vi "Interface.vi"(8 "error in (no error)":errorcluster, 11 "Display Image in":refnum<class "Display Image.lvclass">) -> (0 "error out":errorcluster, 3 "Display Image out":refnum<class "Display Image.lvclass">)   [LabVIEW 2018, in "Display Image.lvclass"]
doc: "This VI presents the interface to view the image acquired by the CCD."
uses:
  Display Image.lvclass
  <vilib>/Utility/inputDevices.llb/mouseAcquire.vi
panel:
  in  "Stop Button":bool
  out "Data:":dbl
  out "Y:":u16
  out "X:":u16
  in  "Histogram":bool
  in  "Logarithmic":bool
  in  "Linear":bool
  out "Stddev":dbl
  out "Mean":dbl
  out "Intensity Graph":dbl[][](graph)
  # "Image Graph"
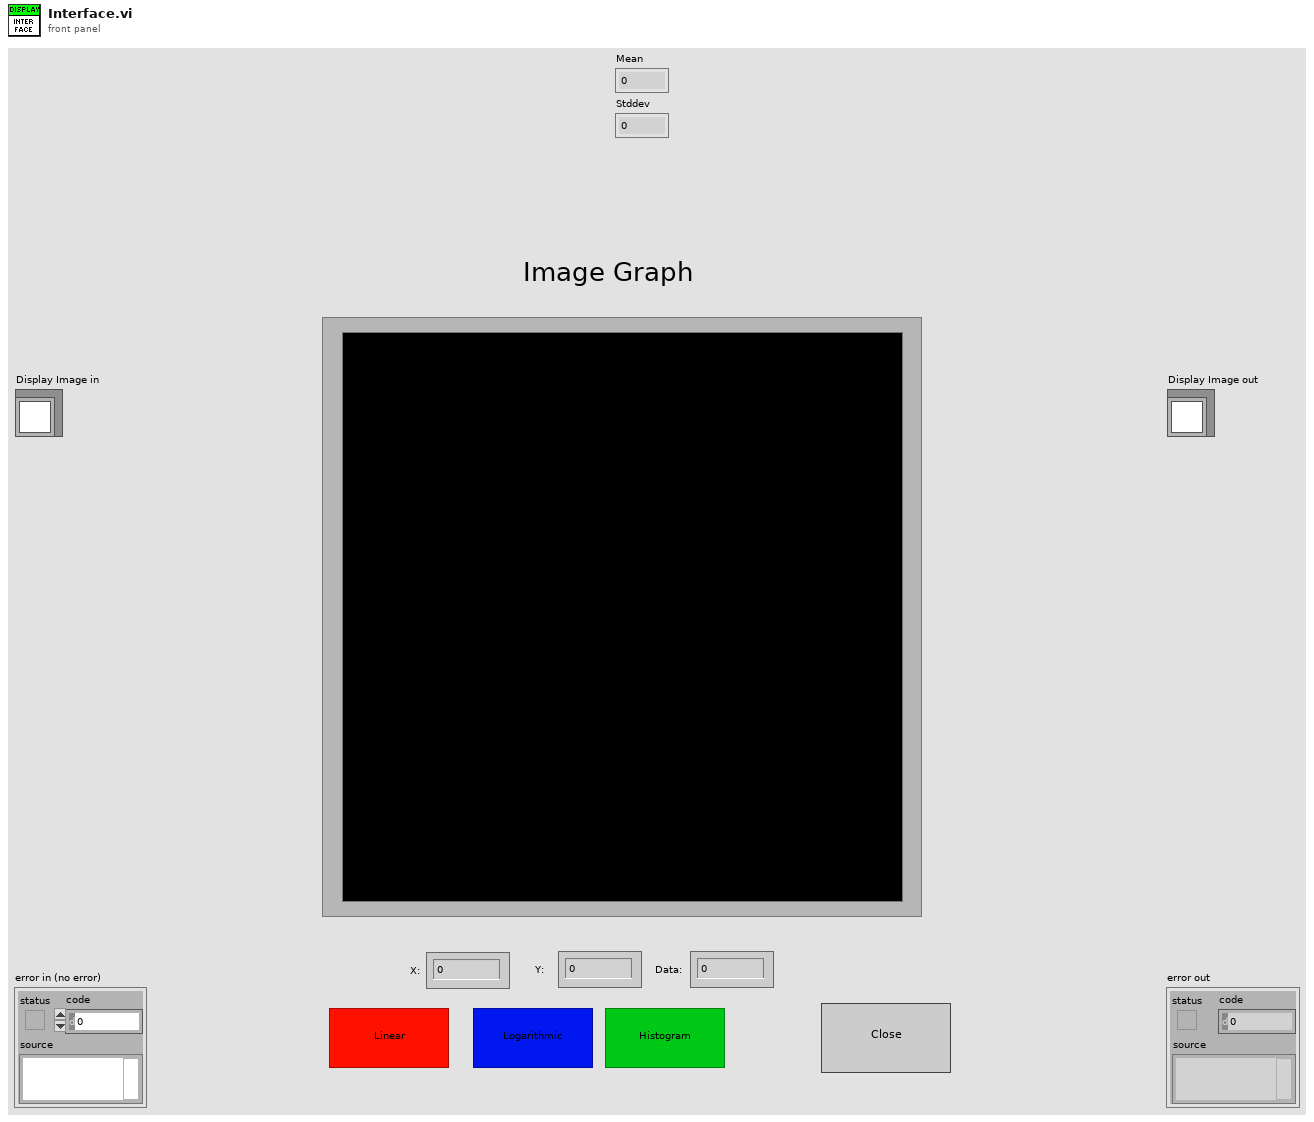
[diagram p1: front panel]
types:
  T1 = cluster{"Horizontal":i32, "Vertical":i32, "Scrolling":i32}
  T2 = typedef "LVPointDoubleTypeDef.ctl" = cluster{"Cursor X":dbl, "Cursor Y":dbl}
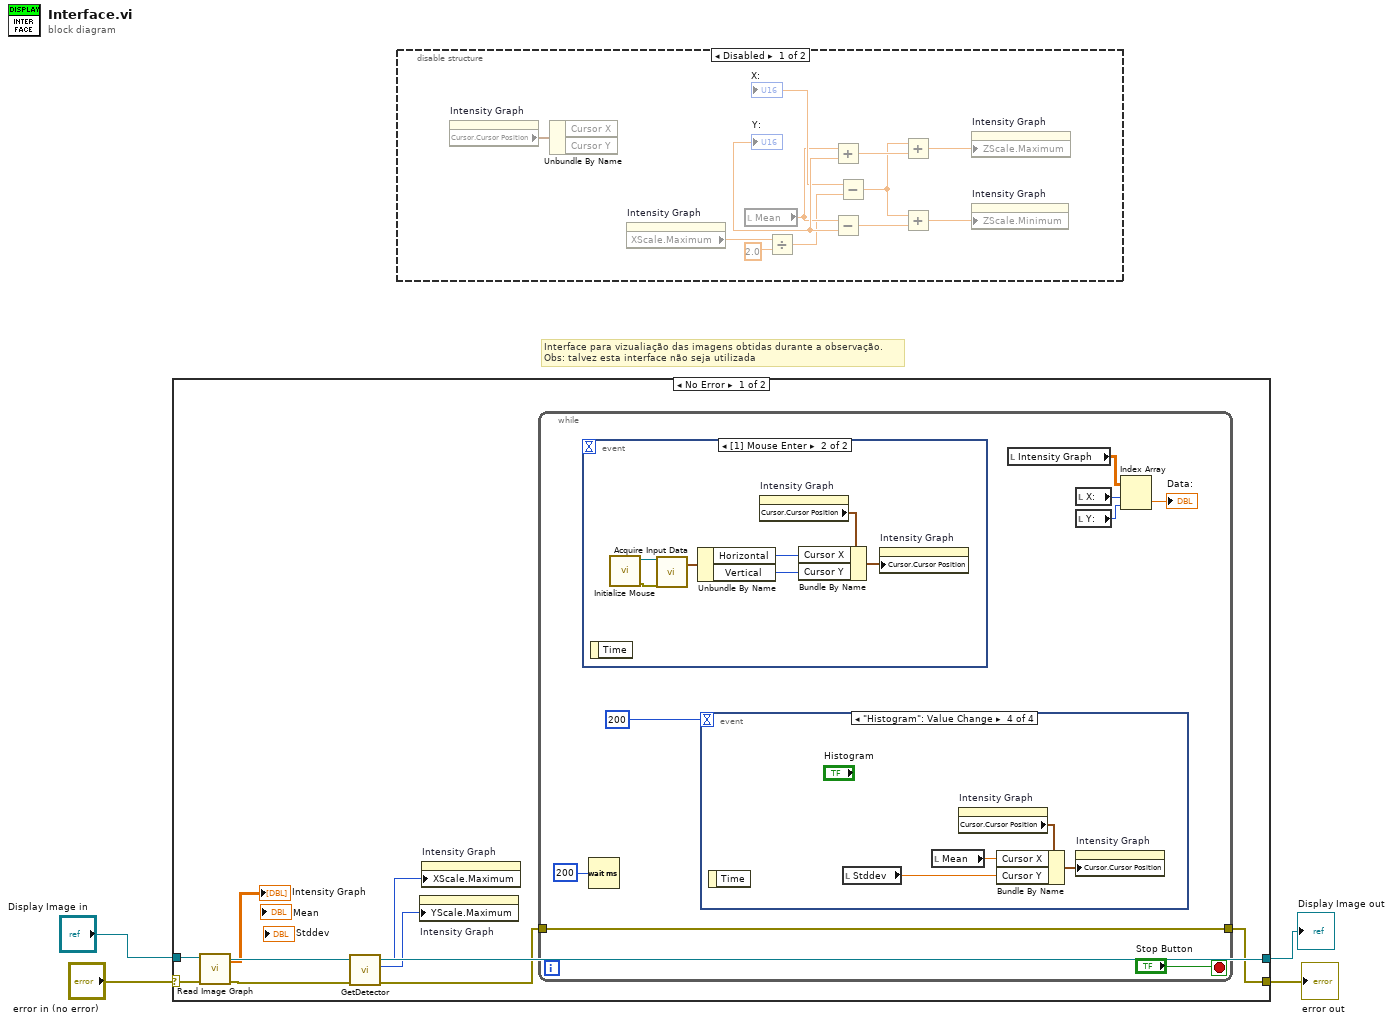
[diagram p0: block diagram]
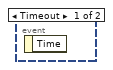
[diagram p3: hidden frame]
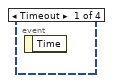
[diagram p4: hidden frame]
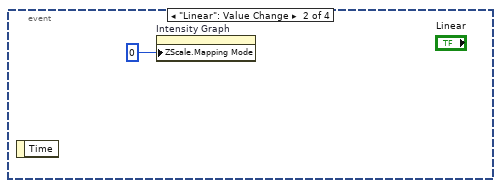
[diagram p5: hidden frame]
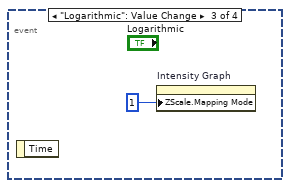
[diagram p6: hidden frame]
diagram:
  # "Interface para vizualiação das imagens obtidas durante a observação. \nObs: talvez esta interface não seja utilizada"
  n1 = case shown="No Error" "error in (no error)" {
    selector: "error in (no error)" -> [w10 w36]
    tunnel: [w5 w36] -> w3
    tunnel: [w12 w35] -> w1
    tunnel: "Display Image in" -> [w13 w35]
    frame No Error {
      n2 = call "Read Image Graph.vi"("error in (no error)"=w10, "Display Image in"=w13) -> ("error out"=w9:errorcluster, "Image Graph"=→"Intensity Graph":dbl[][], "Display Image out"=w12:refnum<class "Display Image.lvclass">)  [unwired: 7 in]
      n3 = call <userlib>:"GetDetector.vi"("error in (no error)"=w9) -> ("error out"=w6:errorcluster, "ypixels"=w8:i32, "xpixels"=w7:i32)  [unwired: 3 in, 1 out]
      n4 = property on="Intensity Graph" class="IntGraph (strict)"("YScale.Maximum"=w8) -> ()  [unwired: 2 in, 2 out]
      n5 = property on="Intensity Graph" class="IntGraph (strict)"("XScale.Maximum"=w7) -> ()  [unwired: 2 in, 2 out]
      n6 = while {
        tunnel: w6 -> [w14]
        tunnel: [w14] -> w5
        stop <- "Stop Button" stop-if-true
        n7 = event shown="[1] Mouse Enter" {
          selector: _ -> [_ _]
          dyn-events: _ -> [_ _]
          timeout: _ -> [_ _]
          event Timeout {
            n8 = event-data() -> ()  [unwired: 1 in, 1 out]
          }
          event Mouse Enter {
            n9 = event-data() -> ()  [unwired: 1 in, 1 out]
            n10 = call <vilib>:"Initialize Mouse.vi"() -> ("error out"=w25:errorcluster, "device ID"=w24:refnum<k1>)  [unwired: 10 in]
            n11 = call-poly <vilib>:"Acquire Input Data.vi"("device ID"=w24, "error in (no error)"=w25) -> ("axis info"=w26:T1)  [unwired: 14 in, 3 out]
            n12 = Unbundle By Name(w26) -> ("Horizontal"=w23:i32, "Vertical"=w22:i32)
            n13 = property on="Intensity Graph" class="IntGraph (strict)"() -> ("Cursor.Cursor Position"=w27:T2)  [unwired: 2 in, 2 out]
            n14 = Bundle By Name(cluster=w27, "Cursor X"=w23, "Cursor Y"=w22) -> (w28:T2)
            n15 = property on="Intensity Graph" class="IntGraph (strict)"("Cursor.Cursor Position"=w28) -> ()  [unwired: 2 in, 2 out]
          }
        }
        n16 = Wait (ms)(milliseconds to wait=u32 200) -> ()  [unwired: 1 out]
        n17 = event shown="[3] \"Histogram\": Value Change" {
          selector: _ -> [_ _ _ _]
          dyn-events: _ -> [_ _ _ _]
          timeout: u32 200 ("milliseconds to wait") -> [_ _ _ _]
          event Timeout {
            n18 = event-data() -> ()  [unwired: 1 in, 1 out]
          }
          event "Linear": Value Change {
            n19 = event-data() -> ()  [unwired: 1 in, 1 out]
            n20 = property on="Intensity Graph" class="IntGraph (strict)"("ZScale.Mapping Mode"=u8 0 ("Z Scale.Mapping Mode")) -> ()  [unwired: 2 in, 2 out]
          }
          event "Logarithmic": Value Change {
            n21 = event-data() -> ()  [unwired: 1 in, 1 out]
            n22 = property on="Intensity Graph" class="IntGraph (strict)"("ZScale.Mapping Mode"=u8 1 ("Z Scale.Mapping Mode")) -> ()  [unwired: 2 in, 2 out]
          }
          event "Histogram": Value Change {
            n23 = event-data() -> ()  [unwired: 1 in, 1 out]
            n24 = local read "Stddev"() -> (w31:dbl)
            n25 = local read "Mean"() -> (w32:dbl)
            n26 = property on="Intensity Graph" class="IntGraph (strict)"() -> ("Cursor.Cursor Position"=w34:T2)  [unwired: 2 in, 2 out]
            n27 = Bundle By Name(cluster=w34, "Cursor X"=w32, "Cursor Y"=w31) -> (w33:T2)
            n28 = property on="Intensity Graph" class="IntGraph (strict)"("Cursor.Cursor Position"=w33) -> ()  [unwired: 2 in, 2 out]
          }
        }
        n29 = local read "Intensity Graph"() -> (w18:dbl[][])
        n30 = local read "X:"() -> (w19:u16)
        n31 = local read "Y:"() -> (w17:u16)
        n32 = Index Array(array=w18, index (row)=w19, index (col)=w17) -> (element=→"Data:":dbl)
      }
    }
    frame Error {
    }
  }
  "error out" <- w3
  "Display Image out" <- w1
  n33 = disable-structure shown="Disabled" {
    frame Disabled {
      n34 = property on="Intensity Graph" class="IntGraph (strict)"() -> ("Cursor.Cursor Position"=w48:T2)  [unwired: 2 in, 2 out]
      n35 = Unbundle By Name(w48) -> ("Cursor X"=w49:dbl, "Cursor Y"=w50:dbl)
      n36 = property on="Intensity Graph" class="IntGraph (strict)"() -> ("XScale.Maximum"=w37:dbl)  [unwired: 2 in, 2 out]
      n37 = local read "Mean"() -> (w40:dbl)
      n38 = Divide(x=w37, y=2.0) -> (x/y=w39:dbl)
      n39 = Add(x=w40) -> (y=w47:dbl, x+y=w42:dbl)
      "Y:" <- w47
      n40 = Subtract(x=w40, y=w47) -> (x-y=w43:dbl)
      n41 = Subtract(y=w39) -> (x=→"X:":dbl, x-y=w41:dbl)
      n42 = Add(x=w41, y=w42) -> (x+y=w44:dbl)
      n43 = Add(x=w41, y=w43) -> (x+y=w45:dbl)
      n44 = property on="Intensity Graph" class="IntGraph (strict)"("ZScale.Maximum"=w44) -> ()  [unwired: 2 in, 2 out]
      n45 = property on="Intensity Graph" class="IntGraph (strict)"("ZScale.Minimum"=w45) -> ()  [unwired: 2 in, 2 out]
    }
    frame Enabled {
    }
  }
